vi "New Protocol.vi"(8 "error in (no error)":errorcluster, 11 "Python Protocol in":refnum<class "Python Protocol.lvclass">) -> (0 "error out":errorcluster, 3 "Python Protocol out":refnum<class "Python Protocol.lvclass">)   [LabVIEW 2012, in "Python Protocol Actor.lvlib" / "Python Protocol.lvclass"]
uses:
  Python Protocol.lvclass
  Python Protocol.lvclass/Python Protocol.ctl
  Read Path.vi
  Read Compiler.vi
  Read Code.vi
  Read New.vi
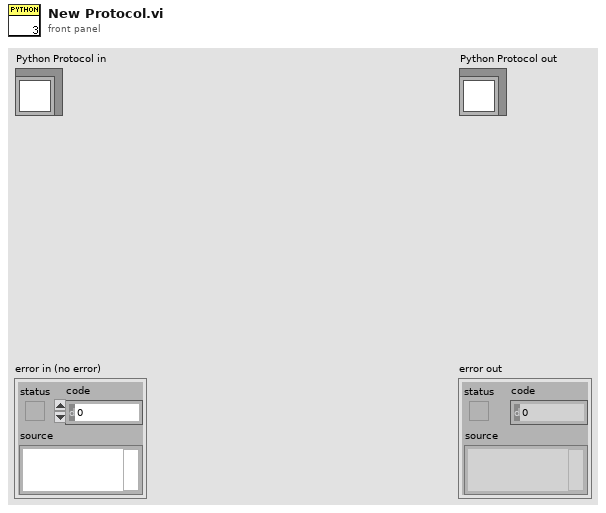
[diagram p1: front panel]
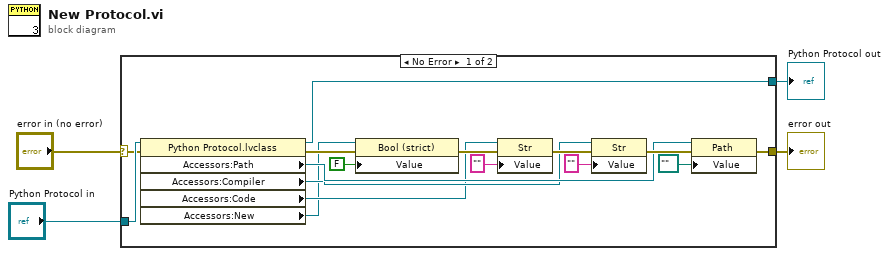
[diagram p0: block diagram]
diagram:
  n1 = case shown="No Error" "error in (no error)" {
    selector: "error in (no error)" -> [w6 w22]
    tunnel: [w5 w22] -> w3
    tunnel: [w12 w21] -> w1
    tunnel: "Python Protocol in" -> [w13 w21]
    frame No Error {
      n2 = property class="Python Protocol.lvclass"(reference=w13, error in=w6) -> (reference out=w12:refnum<class "Python Protocol.lvclass">, error out=w11:errorcluster, "Accessors:Path"=w10:refnum<vi>, "Accessors:Compiler"=w9:refnum<vi>, "Accessors:Code"=w8:refnum<vi>, "Accessors:New"=w7:refnum<vi>)
      n3 = property class="Bool (strict)"(reference=w7, error in=w11, "Value"=FALSE) -> (error out=w20:errorcluster)  [unwired: 1 out]
      n4 = property class="Str"(reference=w8, error in=w20, "Value"="") -> (error out=w18:errorcluster)  [unwired: 1 out]
      n5 = property class="Str"(reference=w9, error in=w18, "Value"="") -> (error out=w15:errorcluster)  [unwired: 1 out]
      n6 = property class="Path"(reference=w10, error in=w15, "Value"=path "") -> (error out=w5:errorcluster)  [unwired: 1 out]
    }
    frame Error {
    }
  }
  "error out" <- w3
  "Python Protocol out" <- w1
